vi "Hyper Cosine fit.vi"(6 "PD width":i32=3 min=3, 8 "PD threshold":dbl=1e-06 format="%.2p", 9 "model and initial parameter input":T2={"a"="a", "b"="b", "c"="c", "d"="d", "ai"=0.0, "bi"=0.0, "ci"=0.0, "di"=0.002} {"di" format="%.3f"; "ci" format="%.3f"; "bi" format="%.3p"; "ai" format="%.2p"}, 10 "Formula":string="a+4*b/(exp(1.7628*(x-c)/d)+exp(-1.7628*(x-c)/d))^2", 11 "Data":cluster{dbl[], dbl[]}(graph)={array[201 elements], array[201 elements]}) -> (0 "std deviation":dbl[](array[numeric])=[9.30078638360989e-23, 3.7103243851581844e-22, 3.6665118721641253e-20, 9.675228079072929e-20], 1 "# of peaks":i32=1, 2 "best fit parameters":dbl[](array[numeric])=[-3.4232233797949633e-23, 1.0000000000000004e-05, 3.766483017079593e-24, 0.002], 3 "Fit":cluster{dbl[], "best nonlinear fit":dbl[]}[](graph))   [LabVIEW 2013]
uses:
  <vilib>/Analysis/Matrix/Datatypes/RealMatrix.ctl
  <vilib>/gmath/NumericalOptimization/Nonlinear Curve Fit LM formula string.vi
  <vilib>/gmath/NI_Gmath.lvlib
  <vilib>/Analysis/NI_AAL_SigProc.lvlib
  <vilib>/Analysis/Matrix/NI_Matrix.lvlib
panel:
  out "R-square":dbl=1.0
  out "residue":cluster{dbl[], dbl[]}(graph)
  out "covariance":T1=[[0.0068443412721599095, -0.003975359172575006, 4.047615105860686e-08, -2.516460911009842], [-0.003975359172575006, 0.1089221180544239, 7.099593891306687e-06, -14.741631824075816], [4.047615105860686e-08, 7.0995938913066875e-06, 1063.6494202794624, -0.0006919743025622302], [-2.5164609110098426, -14.741631824075814, -0.0006919743025622303, 7406.529208760408]] format="%#_5g"
  out "Initial parameters":dbl[](array[numeric])=[0.0, 1.0000000000000004e-05, 0.0, 0.002]
  out "PD peak position":dbl[](array[numeric])
  out "PD Amplitudes":dbl[](array[numeric])=[1.0000000000000004e-05]
  out "PD Locations":dbl[](array[numeric])=[100.00000000000001]
  in  "model description output":T3={"model"="a0+4*b0/(exp(1.7628*(x-c0)/d0)+exp(-1.7628*(x-c0)/d0))^2", "Parameters"=["a0", "b0", "c0", "d0"], "x"="x"}
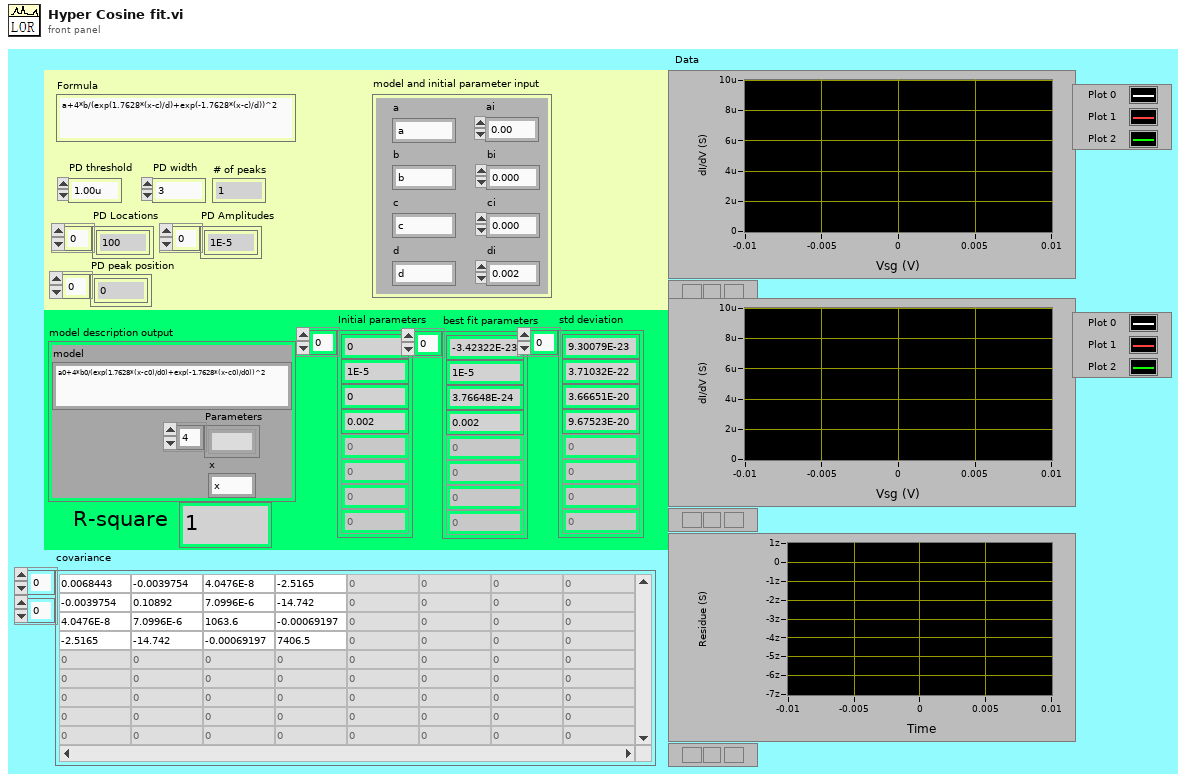
[diagram p1: front panel]
types:
  T1 = typedef "NI_Matrix.lvlib/RealMatrix.ctl" = dbl[][]
  T2 = cluster{"a":string, "b":string, "c":string, "d":string, "ai":dbl, "bi":dbl, "ci":dbl, "di":dbl}
  T3 = cluster{"model":string, "Parameters":string[], "x":string}
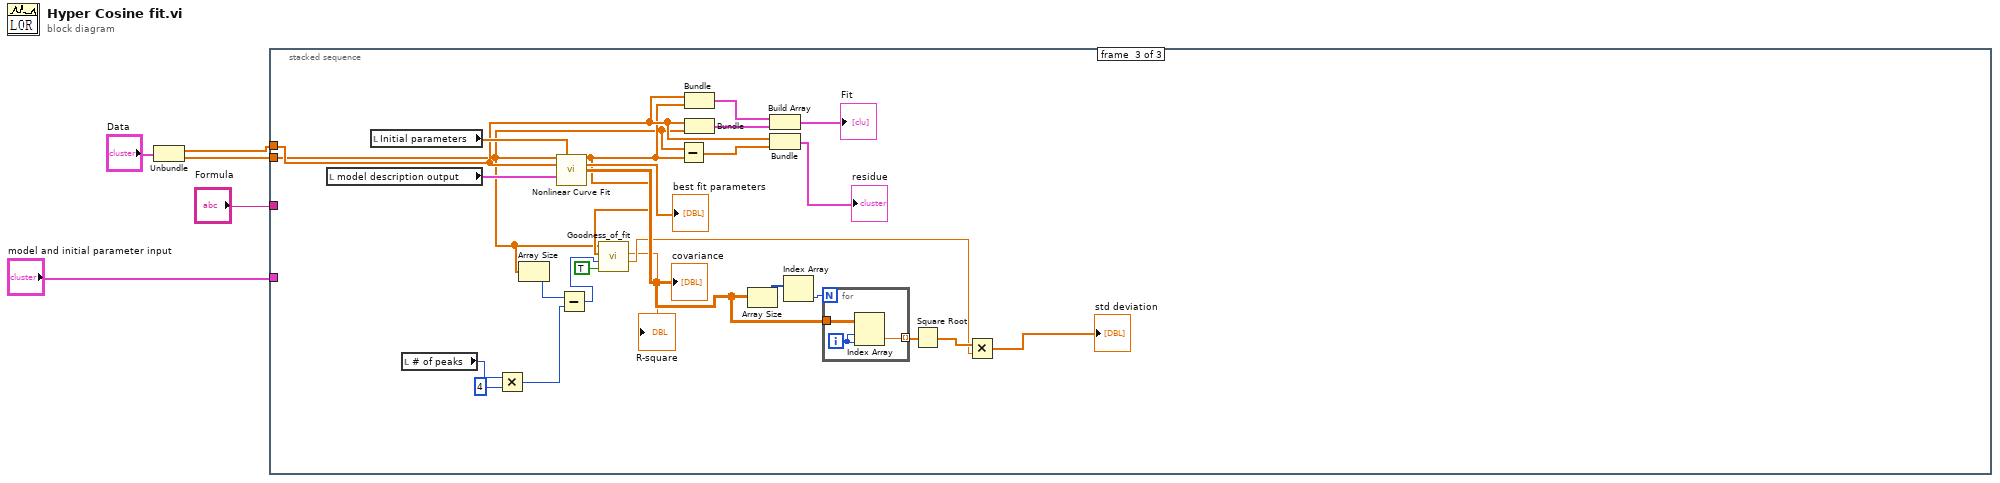
[diagram p0: block diagram]
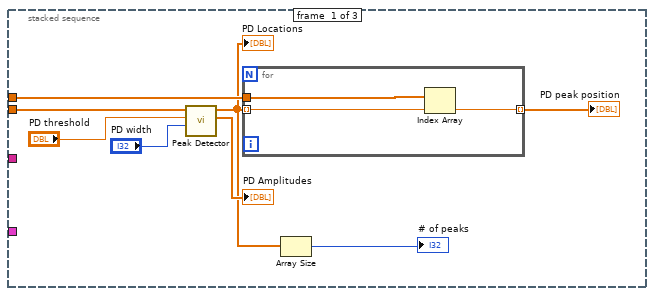
[diagram p2: hidden frame]
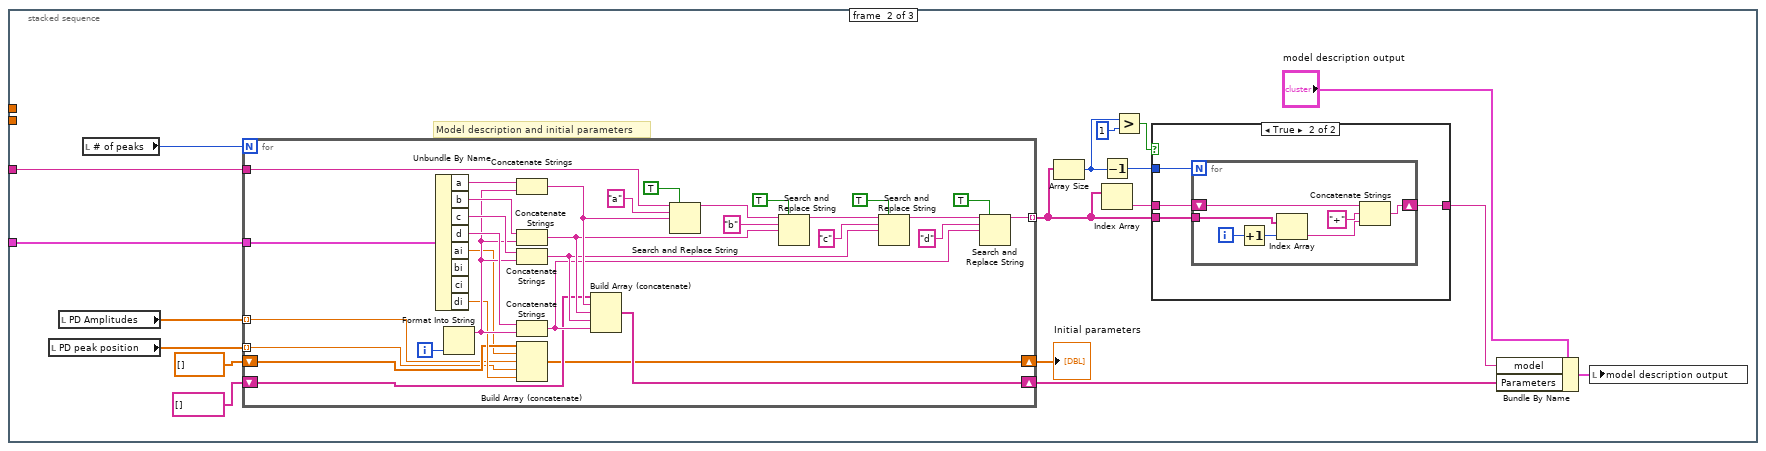
[diagram p3: hidden frame]
diagram:
  n1 = Unbundle("Data") -> (w2:dbl[], w1:dbl[])
  n2 = stacked-sequence {
    tunnel: "Formula" -> [_ w34 _]
    tunnel: "model and initial parameter input" -> [_ w33 _]
    tunnel: w2 -> [w8 _ w96]
    tunnel: w1 -> [w13 _ w88]
    frame #0 {
      n3 = call <vilib>:"Peak Detector.vi"("width"="PD width", "threshold"="PD threshold", "X"=w13) -> ("Amplitudes"=→"PD Amplitudes":dbl[], "Locations"=w7:dbl[])  [unwired: 4 in, 3 out]
      "PD Locations" <- w7
      n4 = for {
        tunnel: w8 -> [w16]
        tunnel: w7 -> [w15] mode=indexing
        tunnel: [w14] -> w6 mode=indexing
        n5 = Index Array(array=w16, index=w15) -> (element=w14:dbl)
      }
      "PD peak position" <- w6
      n6 = Array Size(array=w7) -> (size(s)=→"# of peaks":i32)
    }
    frame #1 {
      # "Model description and initial parameters"
      n7 = local read "PD peak position"() -> (w19:dbl[])
      n8 = local read "PD Amplitudes"() -> (w18:dbl[])
      n9 = local read "# of peaks"() -> (w21:i32)
      n10 = for {
        N: w21 -> [_]
        tunnel: w34 -> [w68]
        tunnel: w33 -> [w77]
        tunnel: [w59] -> w28 mode=indexing
        shift-right: [w54] -> w22
        shift-left: string[] [] -> [w53]
        shift-right: [w51] -> w17
        shift-left: dbl[] [] -> [w50]
        tunnel: w19 -> [w48] mode=indexing
        tunnel: w18 -> [w47] mode=indexing
        i -> [w76]
        n11 = Unbundle By Name(w77) -> ("a"=w75:string, "b"=w74:string, "c"=w73:string, "d"=w72:string, "ai"=w49:dbl, "di"=w52:dbl)  [unwired: 2 out]
        n12 = Format Into String(w76) -> (resulting string=w71:string)  [unwired: 3 in, 1 out]
        n13 = Concatenate Strings(w75, w71) -> (w58:string)
        n14 = Concatenate Strings(w74, w71) -> (w57:string)
        n15 = Concatenate Strings(w73, w71) -> (w56:string)
        n16 = Concatenate Strings(w72, w71) -> (w55:string)
        n17 = Build Array (concatenate)(w50, w49, w47, w48, w52) -> (w51:dbl[])
        n18 = Build Array (concatenate)(w53, w58, w57, w56, w55) -> (w54:string[])
        n19 = Search and Replace String(replace all?=TRUE ("replace all? (F)"), input string=w68, search string="a" ("substring (\"\")"), replace string=w58) -> (result string=w66:string)  [unwired: 4 in, 3 out]
        n20 = Search and Replace String(replace all?=TRUE ("replace all? (F)"), input string=w66, search string="b", replace string=w57) -> (result string=w65:string)  [unwired: 4 in, 3 out]
        n21 = Search and Replace String(replace all?=TRUE ("replace all? (F)"), input string=w65, search string="c", replace string=w56) -> (result string=w64:string)  [unwired: 4 in, 3 out]
        n22 = Search and Replace String(replace all?=TRUE ("replace all? (F)"), input string=w64, search string="d", replace string=w55) -> (result string=w59:string)  [unwired: 4 in, 3 out]
      }
      "Initial parameters" <- w17
      n23 = Array Size(array=w28) -> (size(s)=w30:i32)
      n24 = Decrement(x=w30) -> (x-1=w29:i32)
      n25 = Index Array(array=w28) -> (element=w27:string)  [unwired: 1 in]
      n26 = Greater?(x=w30, y=1) -> (0:w31:bool)
      n27 = case shown="True" w31 {
        tunnel: w28 -> [_ w39]
        tunnel: w29 -> [_ w38]
        tunnel: w27 -> [w35 w37]
        tunnel: [w35 w36] -> w25
        frame False {
        }
        frame True {
          n28 = for {
            N: w38 -> [_]
            tunnel: w39 -> [w43]
            shift-right: [w40] -> w36
            shift-left: w37 -> [w45]
            i -> [w46]
            n29 = Increment(x=w46) -> (x+1=w44:i32)
            n30 = Index Array(array=w43, index=w44) -> (element=w41:string)
            n31 = Concatenate Strings(w45, "+" ("string"), w41) -> (w40:string)
          }
        }
      }
      n32 = Bundle By Name(cluster="model description output", "model"=w25, "Parameters"=w22) -> (w24:T3)
      n33 = local write "model description output"(w24) -> ()
    }
    frame #2 {
      n34 = local read "model description output"() -> (w103:T3)
      n35 = local read "Initial parameters"() -> (w102:dbl[])
      n36 = local read "# of peaks"() -> (w87:i32)
      n37 = Multiply(x=w87, y=4) -> (x*y=w85:i32)
      n38 = Array Size(array=w88) -> (size(s)=w81:i32)
      n39 = call-poly <vilib>:"Nonlinear Curve Fit.vi"("Y"=w88, "initial parameters"=w102, "X"=w96, "model description"=w103) -> ("best nonlinear fit"=w89:dbl[], "best fit parameters"=→"best fit parameters":dbl[], "covariance"=w90:T1)  [unwired: 7 in, 2 out]
      "covariance" <- w90
      n40 = Subtract(x=w81, y=w85) -> (x-y=w80:i32)
      n41 = call <userlib>:"Goodness_of_fit.vi"("Wight=1"=TRUE, "degree of freedom"=w80, "Best Fit"=w89, "Y"=w88) -> ("RMSE"=w83:dbl, "R-square"=→"R-square":dbl)  [unwired: 5 in, 1 out]
      n42 = Subtract(x=w88, y=w89) -> (x-y=w97:dbl[])
      n43 = Bundle(w96, "best nonlinear fit"=w89) -> (w98:cluster{dbl[], "best nonlinear fit":dbl[]})  [unwired: 1 in]
      n44 = Bundle(w96, w88) -> (w99:cluster{dbl[], dbl[]})  [unwired: 1 in]
      n45 = Array Size(array=w90) -> (size(s)=w94:i32[])
      n46 = Build Array(w98, w99) -> (→"Fit":cluster{dbl[], "best nonlinear fit":dbl[]}[])
      n47 = Bundle(w96, w97) -> (→"residue":cluster{dbl[], dbl[]})  [unwired: 1 in]
      n48 = Index Array(array=w94) -> (element=w93:i32)  [unwired: 1 in]
      n49 = for {
        N: w93 -> [_]
        tunnel: w90 -> [w106]
        tunnel: [w104] -> w92 mode=indexing
        i -> [w105]
        n50 = Index Array(array=w106, index (row)=w105, index (col)=w105) -> (element=w104:dbl)
      }
      n51 = Square Root(x=w92) -> (sqrt(x)=w91:dbl[])
      n52 = Multiply(x=w91, y=w83) -> (x*y=→"std deviation":dbl[])
    }
  }
